vi "Asylum_Driver_XYMetersToVoltage.vi"(8 "error in (no error)":errorcluster, 9 "Y Coordinate":dbl, 10 "X Coordinate":dbl, 11 "Application":refnum<k7>) -> (0 "error out":errorcluster, 1 "Y Voltage":dbl, 2 "X Voltage":dbl, 3 "Application":refnum<k7>)   [LabVIEW 2019]
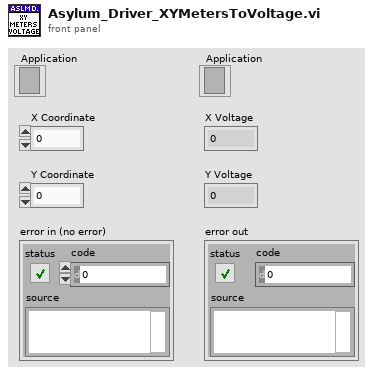
[diagram p1: front panel]
types:
  T1 = cluster{"XLVDT Sens":dbl, "YLVDT Sens":dbl, "XLVDT Offset":dbl, "YLVDT Offset":dbl}
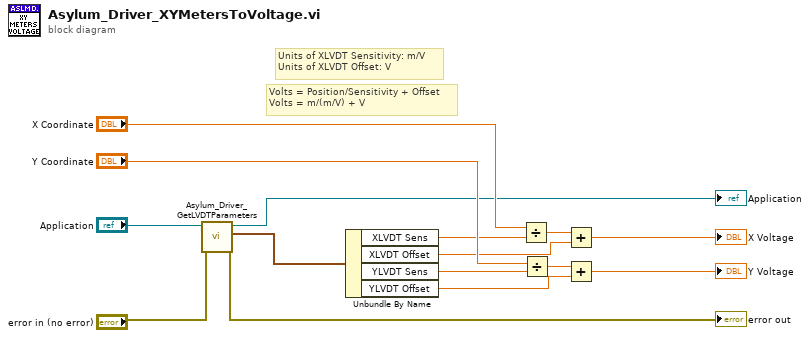
[diagram p0: block diagram]
diagram:
  # "Units of XLVDT Sensitivity: m/V\nUnits of XLVDT Offset: V"
  # "Volts = Position/Sensitivity + Offset\nVolts = m/(m/V) + V"
  n1 = call "Asylum_Driver_GetLVDTParameters.vi"("error in (no error)"="error in (no error)", "Application"="Application") -> ("error out"=→"error out":errorcluster, "LVDT Parameters"=w1:T1, "Application"=→"Application":refnum<k7>)  [unwired: 7 in]
  n2 = Unbundle By Name(w1) -> ("XLVDT Sens"=w2:dbl, "XLVDT Offset"=w4:dbl, "YLVDT Sens"=w3:dbl, "YLVDT Offset"=w7:dbl)
  n3 = Divide(x="X Coordinate", y=w2) -> (x/y=w5:dbl)
  n4 = Divide(x="Y Coordinate", y=w3) -> (x/y=w6:dbl)
  n5 = Add(x=w5, y=w4) -> (x+y=→"X Voltage":dbl)
  n6 = Add(x=w6, y=w7) -> (x+y=→"Y Voltage":dbl)
